vi "NicmosSetFilterWheel.vi"(0 "error in (no error)":errorcluster caption="entrée d'erreur", 5 "Filter":i32(ring) items=["1", "2", "3", "4", "5", "6", "7", "8", "9", "10", "11", "12"], 6 "Offset":i16(slide) scale=-500.0..500.0, 7 "Initialize":bool) -> (3 "error out":errorcluster caption="sortie d'erreur")   [LabVIEW 2009]
uses:
  NicmosGlobal.vi
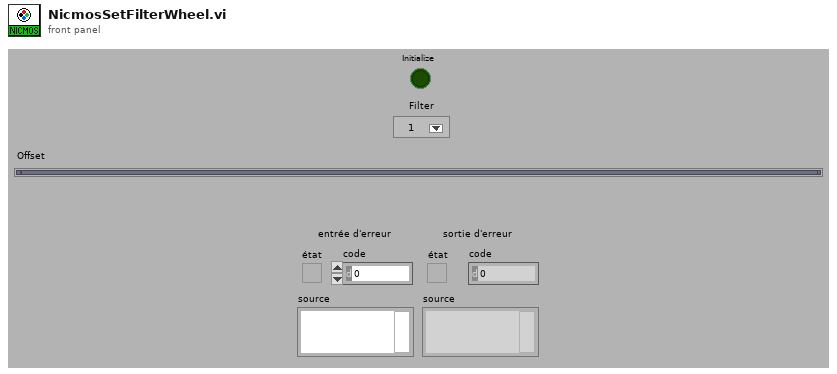
[diagram p1: front panel]
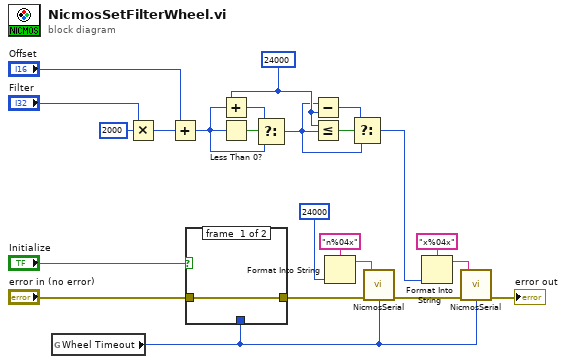
[diagram p0: block diagram]
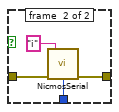
[diagram p2: hidden frame]
diagram:
  w13 = i16 24000 ("x")
  n1 = global read "NicmosGlobal.vi" "Wheel Timeout"() -> (w2:i32)
  n2 = Multiply(x="Filter", y=i16 2000) -> (x*y=w20:i32)
  n3 = Add(x="Offset", y=w20) -> (x+y=w16:i32)
  n4 = case shown="True" "Initialize" {
    tunnel: [w24 w26] -> w5
    tunnel: "error in (no error)" -> [w24 w28]
    tunnel: w2 -> [_ w25]
    frame #0 {
    }
    frame #1 {
      n5 = call "NicmosSerial.vi"("error in"=w28, "timeout (10sec)"=w25, "Command"="i" ("Question L")) -> ("error out"=w26:errorcluster)  [unwired: 2 in, 1 out]
    }
  }
  n6 = Add(x=w13, y=w16) -> (x+y=w17:i32)
  n7 = Less Than 0?(x=w16) -> (x < 0?=w18:bool)
  n8 = Select(t=w17, s=w18, f=w16) -> (s? t:f=w12:i32)
  n9 = Subtract(x=w12, y=w13) -> (x-y=w14:i32)
  n10 = Less Or Equal?(x=w13, y=w12) -> (x <= y?=w15:bool)
  n11 = Format Into String(format string="n%04x" ("Question L"), 24000) -> (resulting string=w8:string)  [unwired: 2 in, 1 out]
  n12 = Select(t=w14, s=w15, f=w12) -> (s? t:f=w11:i32)
  n13 = call "NicmosSerial.vi"("error in"=w5, "timeout (10sec)"=w2, "Command"=w8) -> ("error out"=w6:errorcluster)  [unwired: 2 in, 1 out]
  n14 = Format Into String(format string="x%04x" ("Question L"), w11) -> (resulting string=w3:string)  [unwired: 2 in, 1 out]
  n15 = call "NicmosSerial.vi"("error in"=w6, "timeout (10sec)"=w2, "Command"=w3) -> ("error out"=→"error out":errorcluster)  [unwired: 2 in, 1 out]
